vi "As Task Kind.vi"(1 "Sensor Type":T1) -> (0 "DAQmx Task prefix":string)   [LabVIEW 2021, in "Load Frame.lvlib"]
doc: "Convert the Application's typedef value for a sensor type to the corresponding DAQmx Task kind (like AI or Counter)."
uses:
  Load Frame.lvlib
  Acquisition/Sensor Type.ctl
  Acquisition/Acquisition.lvlib
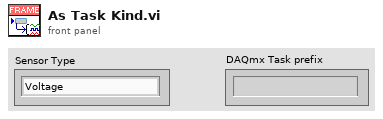
[diagram p1: front panel]
types:
  T1 = typedef "Acquisition.lvlib/Sensor Type.ctl" = enum16{"Voltage", "Load", "Pressure", "Encoder"}
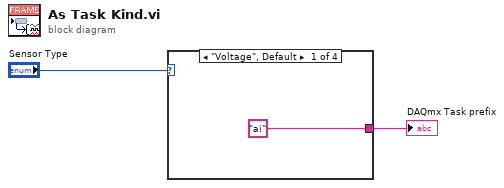
[diagram p0: block diagram]
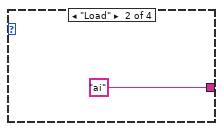
[diagram p2: hidden frame]
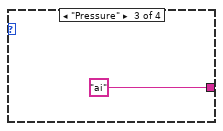
[diagram p3: hidden frame]
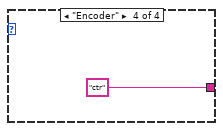
[diagram p4: hidden frame]
diagram:
  n1 = case shown="\"Voltage\", Default" "Sensor Type" {
    tunnel: ["ai" ("DAQmx Task prefix") "ai" ("DAQmx Task prefix") "ai" ("DAQmx Task prefix") "ctr" ("DAQmx Task prefix")] -> w1
    frame "Voltage", Default {
    }
    frame "Load" {
    }
    frame "Pressure" {
    }
    frame "Encoder" {
    }
  }
  "DAQmx Task prefix" <- w1
